vi "Front Panel - Title--Const.vi"() -> (3 "Window Title":string)   [LabVIEW 2017, in "DTacq Plot Display Library.lvlib"]
uses:
  DTacq Plot Display Library.lvlib
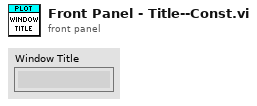
[diagram p1: front panel]
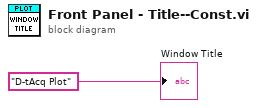
[diagram p0: block diagram]
diagram:
  "Window Title" <- "D-tAcq Plot" ("Front Panel Window:Title")
